vi "DVRTFIFO.vi"() -> ()   [LabVIEW 2013]
uses:
  dtype.ctl
panel:
  out "Array":T1[](array[typedef])
  out "x = y?":bool
  out "dt":dbl
  in  "base size":i32=10000
  in  "count":i32=100
  in  "QCnt":u32=10
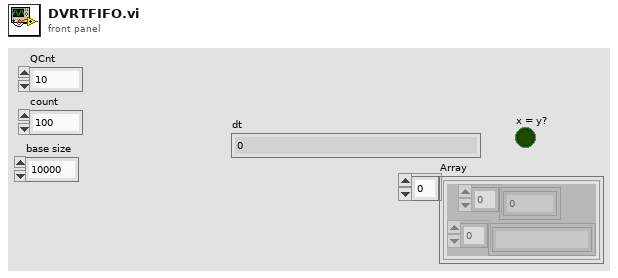
[diagram p1: front panel]
types:
  T1 = typedef "dtype.ctl" = cluster{dbl[], string[]}
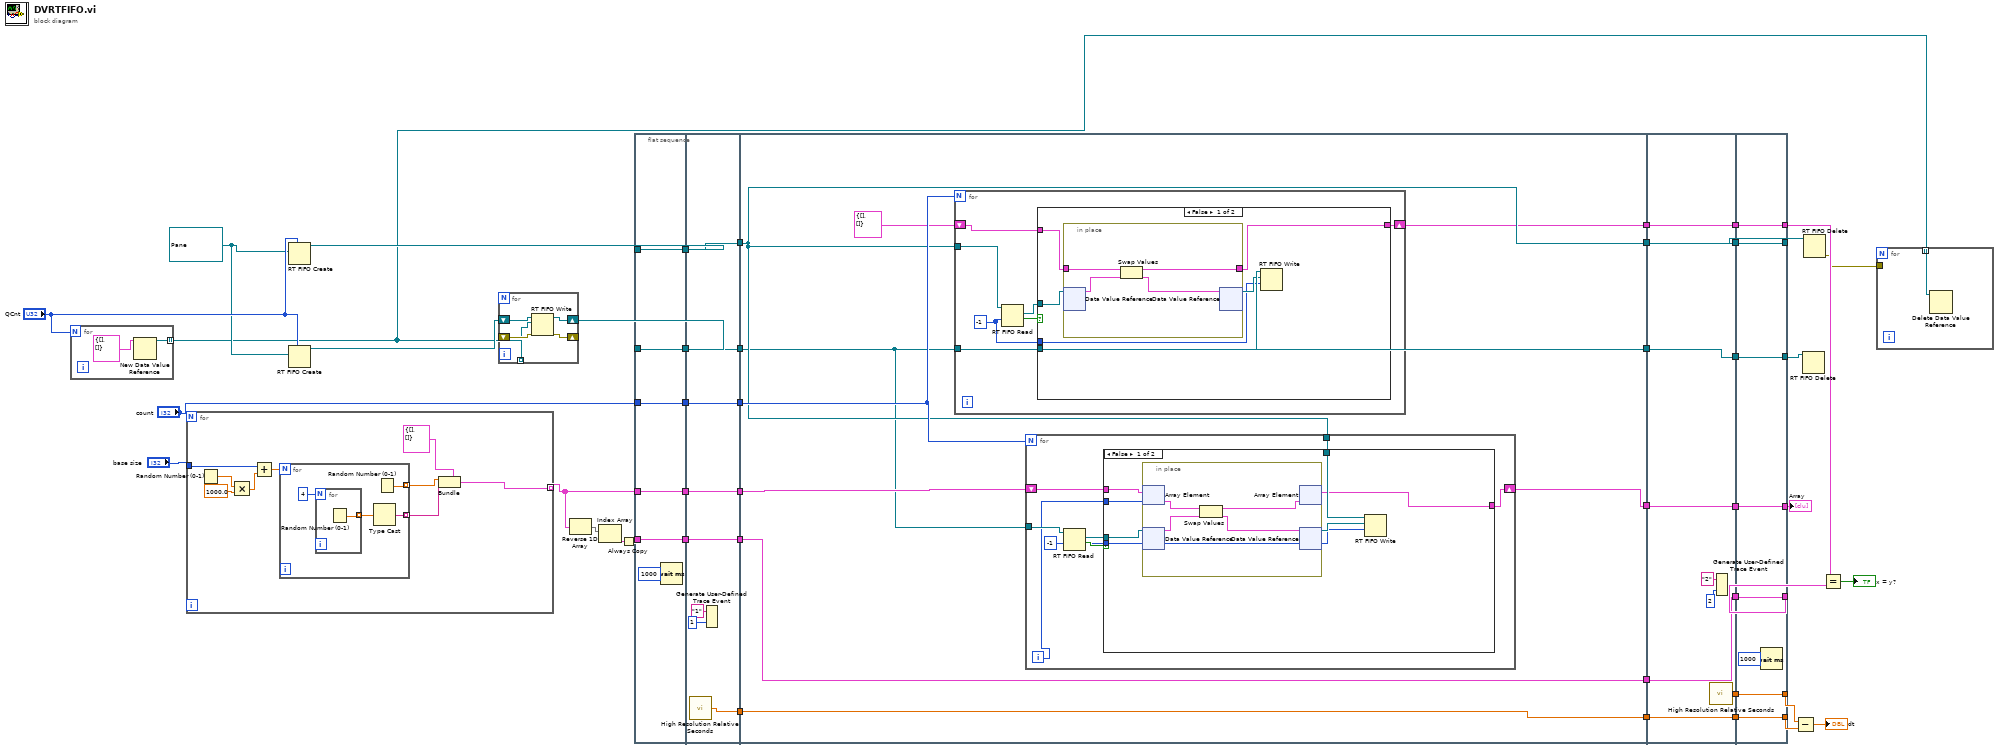
[diagram p0: block diagram]
diagram:
  w21 = refnum<data-value> refnum ("data value reference")
  n1 = for {
    N: "QCnt" -> [_]
    tunnel: [w47] -> w15 mode=indexing
    n2 = New Data Value Reference(data value=T1 {[], []}) -> (data value reference=w47:refnum<data-value>)  [unwired: 1 in, 1 out]
  }
  n3 = for {
    N: "count" -> [_]
    tunnel: [w52] -> w29 mode=indexing
    tunnel: "base size" -> [w51]
    n4 = Random Number (0-1)() -> (number: 0 to 1=w57:dbl)
    n5 = Multiply(x=w57, y=1000.0) -> (x*y=w55:dbl)
    n6 = Add(x=w51, y=w55) -> (x+y=w54:dbl)
    n7 = for {
      N: w54 -> [_]
      tunnel: [w61] -> w50 mode=indexing
      tunnel: [w58] -> w49 mode=indexing
      n8 = for {
        N: 4 -> [_]
        tunnel: [w62] -> w59 mode=indexing
        n9 = Random Number (0-1)() -> (number: 0 to 1=w62:dbl)
      }
      n10 = Type Cast(x=w59) -> (*(type *) &x=w58:string)  [unwired: 1 in]
      n11 = Random Number (0-1)() -> (number: 0 to 1=w61:dbl)
    }
    n12 = Bundle(cluster=T1 {[], []}, w50, w49) -> (w52:T1)
  }
  n13 = RT FIFO Create(1:w21, 4:"QCnt") -> (8:w20:refnum<k33>)  [unwired: 6 in, 2 out]
  n14 = RT FIFO Create(1:w21, 4:"QCnt") -> (8:w18:refnum<k33>)  [unwired: 6 in, 2 out]
  n15 = for {
    shift-right: [w65] -> w19
    shift-left: w18 -> [w67]
    shift-right: [w64] -> _
    shift-left: _ -> [w66]
    tunnel: w15 -> [w63] mode=indexing
    n16 = RT FIFO Write(0:w67, 1:w63, 3:w66) -> (8:w65:refnum<k33>, 11:w64:errorcluster)  [unwired: 2 in, 2 out]
  }
  n17 = Reverse 1D Array(array=w29) -> (reversed array=w30:T1[])
  n18 = Index Array(array=w30) -> (element=w13:T1)  [unwired: 1 in]
  n19 = Always Copy(1:w13) -> (0:w26:T1)
  n20 = flat-sequence {
    tunnel: w26 -> [w69]
    tunnel: w29 -> [w70]
    tunnel: "count" -> [w71]
    tunnel: w19 -> [w72]
    tunnel: w20 -> [w73]
    tunnel: [w73] -> w12
    tunnel: [w72] -> w11
    tunnel: [w71] -> w10
    tunnel: [w70] -> w9
    tunnel: [w69] -> w8
    tunnel: [w81] -> w44
    tunnel: [w80] -> w39
    tunnel: [w79] -> w37
    tunnel: [w78] -> w34
    tunnel: [w77] -> w32
    tunnel: [w76] -> w27
    tunnel: w12 -> [w80]
    tunnel: w11 -> [w79]
    tunnel: w10 -> [w78]
    tunnel: w9 -> [w77]
    tunnel: w8 -> [w76]
    tunnel: w44 -> [w90]
    tunnel: [w90] -> w43
    tunnel: [w87] -> w40
    tunnel: w39 -> [w87]
    tunnel: [w85] -> w38
    tunnel: w37 -> [w85]
    tunnel: w34 -> [w89]
    tunnel: w32 -> [w88]
    tunnel: [w84] -> w31
    tunnel: [w83] -> w28
    tunnel: w27 -> [w83]
    tunnel: [w82] -> w17
    tunnel: w43 -> [w136]
    tunnel: w40 -> [w135]
    tunnel: w38 -> [w134]
    tunnel: w31 -> [w133]
    tunnel: w28 -> [w132]
    tunnel: w17 -> [w129]
    tunnel: [w137] -> w7
    tunnel: [w136] -> w6
    tunnel: [w135] -> w5
    tunnel: [w134] -> w4
    tunnel: [w133] -> w3
    tunnel: [w132] -> w2
    tunnel: [w129] -> w1
    tunnel: [w139] -> w14
    tunnel: [w140] -> w25
    tunnel: [w141] -> w24
    tunnel: [w142] -> w35
    tunnel: [w143] -> w36
    tunnel: [w144] -> w42
    tunnel: [w145] -> w45
    tunnel: w7 -> [w145]
    tunnel: w6 -> [w144]
    tunnel: w5 -> [w143]
    tunnel: w4 -> [w142]
    tunnel: w3 -> [w141]
    tunnel: w2 -> [w140]
    tunnel: w1 -> [w139]
    frame #0 {
      n21 = Wait (ms)(milliseconds to wait=u32 1000) -> ()  [unwired: 1 out]
    }
    frame #1 {
      n22 = call <vilib>:"High Resolution Relative Seconds.vi"() -> ("relative seconds"=w81:dbl)
      n23 = Generate User-Defined Trace Event(1:1 ("trace integer"), 2:"1" ("trace string")) -> ()
    }
    frame #2 {
      n24 = for {
        N: w89 -> [_]
        tunnel: w87 -> [w117]
        shift-right: [w114] -> w84
        shift-left: T1 {[], []} -> [w115]
        tunnel: w85 -> [w112]
        w111 = -1 ("timeout in ms (0)")
        n25 = RT FIFO Read(0:w117, 2:w111) -> (9:w113:refnum<data-value>, 10:w116:bool)  [unwired: 2 in, 3 out]
        n26 = case shown="False" w116 {
          tunnel: w113 -> [w122 _]
          tunnel: w115 -> [w120 w128]
          tunnel: [w119 w128] -> w114
          tunnel: w112 -> [w123 _]
          tunnel: w111 -> [w118 _]
          frame False {
            n27 = in-place {
              in-place-border: w120 -> [w126]
              in-place-border: [w124] -> w119
              n28 = in-place-dvr #1(w122) -> (w127:T1)  [unwired: 1 out]
              n29 = Swap Values(12:w126, 14:w127) -> (1:w124:T1, 3:w125:T1)  [unwired: 1 in]
              n30 = in-place-dvr #1(w125) -> (w121:refnum<data-value>)  [unwired: 1 out]
            }
            n31 = RT FIFO Write(0:w123, 1:w121, 2:w118) -> ()  [unwired: 2 in, 4 out]
          }
          frame True {
          }
        }
      }
      n32 = for {
        N: w89 -> [_]
        tunnel: w85 -> [w98]
        tunnel: w87 -> [w94]
        shift-right: [w92] -> w82
        shift-left: w88 -> [w95]
        i -> [w91]
        w93 = -1 ("timeout in ms (0)")
        n33 = RT FIFO Read(0:w98, 2:w93) -> (9:w96:refnum<data-value>, 10:w97:bool)  [unwired: 2 in, 3 out]
        n34 = case shown="False" w97 {
          tunnel: w96 -> [w104 _]
          tunnel: w95 -> [w101 w110]
          tunnel: w94 -> [w105 _]
          tunnel: w93 -> [w102 _]
          tunnel: [w100 w110] -> w92
          tunnel: w91 -> [w99 _]
          frame False {
            n35 = in-place {
              n36 = in-place-array #2(w101, w99) -> (w107:T1)
              n37 = in-place-dvr #3(w104) -> (w109:T1)  [unwired: 1 out]
              n38 = Swap Values(12:w107, 14:w109) -> (1:w106:T1, 3:w108:T1)  [unwired: 1 in]
              n39 = in-place-array #2(w106) -> (w100:T1[])  [unwired: 1 out]
              n40 = in-place-dvr #3(w108) -> (w103:refnum<data-value>)  [unwired: 1 out]
            }
            n41 = RT FIFO Write(0:w105, 1:w103, 2:w102) -> ()  [unwired: 2 in, 4 out]
          }
          frame True {
          }
        }
      }
    }
    frame #3 {
      n42 = call <vilib>:"High Resolution Relative Seconds.vi"() -> ("relative seconds"=w137:dbl)
      n43 = Generate User-Defined Trace Event(1:2 ("trace integer"), 2:"2" ("trace string")) -> ()
    }
    frame #4 {
      n44 = Wait (ms)(milliseconds to wait=u32 1000) -> ()  [unwired: 1 out]
    }
  }
  n45 = Subtract(x=w45, y=w42) -> (x-y=→"dt":dbl)
  n46 = RT FIFO Delete(0:w35) -> ()  [unwired: 2 in, 1 out]
  n47 = RT FIFO Delete(0:w36) -> (11:w16:errorcluster)  [unwired: 2 in]
  n48 = Equal?(x=w24, y=w25) -> (x = y?=→"x = y?":bool)
  n49 = for {
    tunnel: w16 -> [_]
    tunnel: w15 -> [w146] mode=indexing
    n50 = Delete Data Value Reference(data value reference=w146) -> ()  [unwired: 1 in, 2 out]
  }
  "Array" <- w14
